vi "Go Home.vi"() -> ()   [LabVIEW 2017]
uses:
  Go Home State type def.ctl
panel:
  in  "stop":bool
  out "Motor Status":cluster{"Homing Freq":dbl, "Homing Duty %":dbl} {"Homing Duty %" format="%#_13g"; "Homing Freq" format="%#_13g"}
  in  "Homing Duty %":dbl format="%#_13g"
  in  "Homing Freq":dbl format="%#_13g"
  in  "error in (no error)":errorcluster
  out "error out":errorcluster
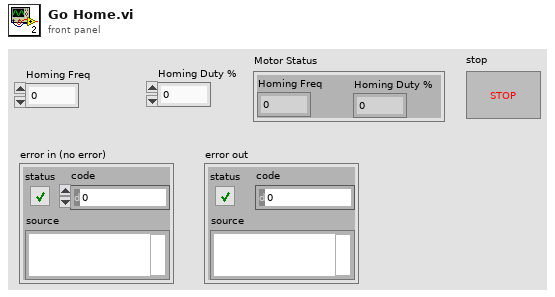
[diagram p1: front panel]
types:
  T1 = typedef "Go Home State type def.ctl" = enum16{"Stop Motor", "Read Input", "Drive Y", "Drive X"}
  T2 = typedef "Encoder Count Direction Enum.ctl" = enum16{"Counting Up", "Counting Down"}
  T3 = cluster{"Y-axis rev count":dbl, "Y-axis distance":dbl, "X-axis rev count":dbl, "X-axis distance":dbl, "Y-axis direction":T2, "X-axis direction":T2, "X-counter val":i32, "Y-counter val":i32}
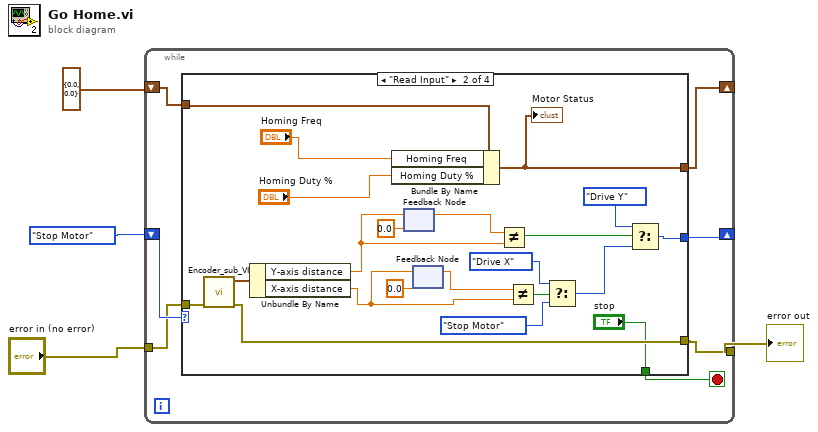
[diagram p0: block diagram]
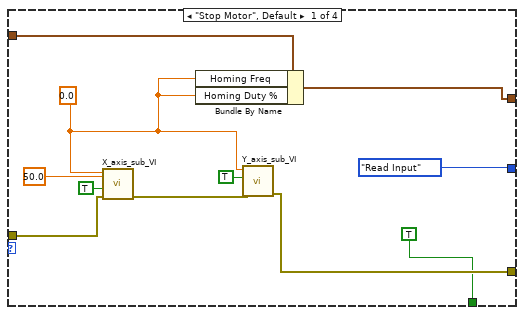
[diagram p2: hidden frame]
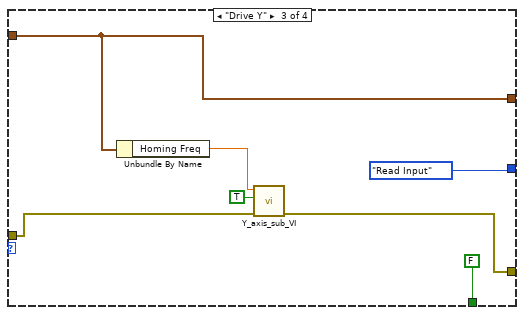
[diagram p3: hidden frame]
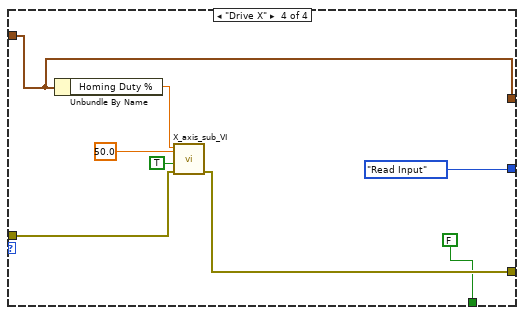
[diagram p4: hidden frame]
diagram:
  n1 = while {
    tunnel: "error in (no error)" -> [w7]
    tunnel: [w6] -> w3
    shift-right: [w8] -> _
    shift-left: Go_Home_State_type_def."Stop Motor" -> [w11]
    shift-right: [w9] -> _
    shift-left: cluster{"Homing Freq":dbl, "Homing Duty %":dbl} {"Homing Freq"=0.0, "Homing Duty %"=0.0} ("Cluster 2") -> [w10]
    stop <- w5 stop-if-true
    n2 = case shown="\"Read Input\"" w11 {
      tunnel: w10 -> [w22 w42 w44 w53]
      tunnel: [w21 w40 w44 w53] -> w9
      tunnel: [Go_Home_State_type_def."Read Input" w30 Go_Home_State_type_def."Read Input" Go_Home_State_type_def."Read Input"] -> w8
      tunnel: w7 -> [w18 w25 w48 w56]
      tunnel: [w19 w24 w47 w55] -> w6
      tunnel: [TRUE "stop" FALSE ("stop") FALSE ("stop")] -> w5
      frame "Stop Motor", Default {
        w17 = 0.0
        n3 = call "X_axis_sub_VI.vi"("error in (no error)"=w18, "FWD/RVS"=TRUE, "Frequency"=50.0, "Duty Cycle %"=w17) -> ("error out"=w20:errorcluster)  [unwired: 7 in]
        n4 = Bundle By Name(cluster=w22, "Homing Freq"=w17, "Homing Duty %"=w17) -> (w21:cluster{"Homing Freq":dbl, "Homing Duty %":dbl})
        n5 = call "Y_axis_sub_VI.vi"("error in (no error)"=w20, "FWD/RVS"=TRUE, "Frequency"=w17) -> ("error out"=w19:errorcluster)  [unwired: 8 in]
      }
      frame "Read Input" {
        n6 = call "Encoder_sub_VI.vi"("error in (no error)"=w25) -> ("error out"=w24:errorcluster, "Encoder Output"=w39:T3)  [unwired: 9 in]
        n7 = Unbundle By Name(w39) -> ("Y-axis distance"=w36:dbl, "X-axis distance"=w33:dbl)
        n8 = Bundle By Name(cluster=w42, "Homing Freq"="Homing Freq", "Homing Duty %"="Homing Duty %") -> (w40:cluster{"Homing Freq":dbl, "Homing Duty %":dbl})
        "Motor Status" <- w40
        n9 = feedback-in #1(w36) -> ()
        n10 = feedback #1(0.0 ("Y-axis distance")) -> (w37:dbl)
        n11 = feedback #2(0.0 ("Y-axis distance")) -> (w35:dbl)
        n12 = feedback-in #2(w33) -> ()
        n13 = Not Equal?(x=w37, y=w36) -> (x != y?=w32:bool)
        n14 = Not Equal?(x=w35, y=w33) -> (x != y?=w29:bool)
        n15 = Select(t=Go_Home_State_type_def."Drive X", s=w29, f=Go_Home_State_type_def."Stop Motor") -> (s? t:f=w28:T1)
        n16 = Select(t=Go_Home_State_type_def."Drive Y", s=w32, f=w28) -> (s? t:f=w30:T1)
      }
      frame "Drive Y" {
        n17 = Unbundle By Name(w44) -> ("Homing Freq"=w45:dbl)
        n18 = call "Y_axis_sub_VI.vi"("error in (no error)"=w48, "FWD/RVS"=TRUE, "Frequency"=w45) -> ("error out"=w47:errorcluster)  [unwired: 8 in]
      }
      frame "Drive X" {
        n19 = Unbundle By Name(w53) -> ("Homing Duty %"=w54:dbl)
        n20 = call "X_axis_sub_VI.vi"("error in (no error)"=w56, "FWD/RVS"=TRUE, "Frequency"=50.0, "Duty Cycle %"=w54) -> ("error out"=w55:errorcluster)  [unwired: 7 in]
      }
    }
  }
  "error out" <- w3
